vi "Append Report Text (str).vi"(0 "report in":refnum<class "NI_Standard Report.lvclass">, 1 "MS Office parameters":T1, 2 "format string (%.3f)":string="%.3f", 7 "text":string, 9 "append on new line? (F)":bool, 11 "error in (no error)":errorcluster) -> (4 "report out":refnum<class "NI_Standard Report.lvclass">, 8 "start out (Word)":i32, 10 "end out (Word)":i32, 15 "error out":errorcluster)   [LabVIEW 2015, in "NI_Standard Report.lvclass"]
doc: "Appends text to the selected report."
uses:
  <vilib>/Utility/NIReport.llb/Standard Report/NI_Standard Report.lvclass
  <vilib>/Utility/NIReport.llb/Standard Report/NI_Standard Report.lvclass/NI_Standard Report.ctl
  <vilib>/Utility/NIReport.llb/NI_ReportGenerationCore.lvlib
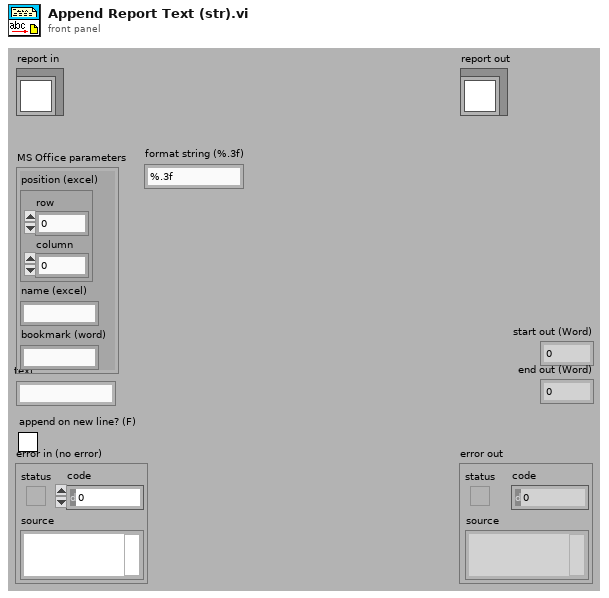
[diagram p1: front panel]
types:
  T1 = cluster{"position (excel)":cluster{"row":i32, "column":i32}, "name (excel)":string, "bookmark (word)":string}
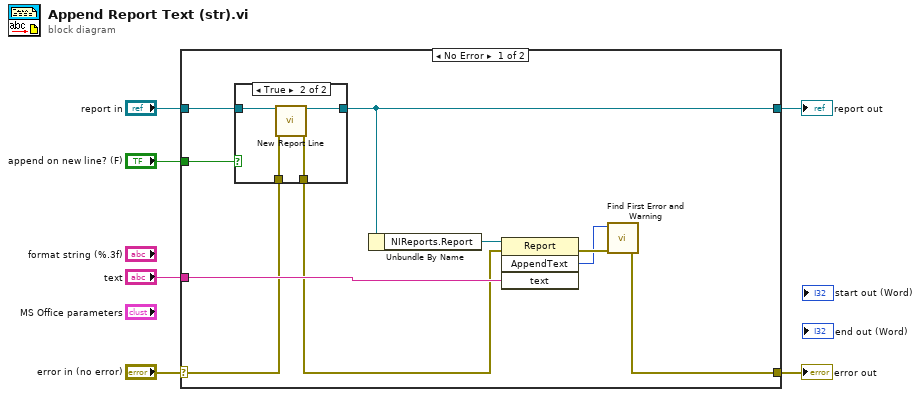
[diagram p0: block diagram]
diagram:
  n1 = case shown="No Error" "error in (no error)" {
    selector: "error in (no error)" -> [w8 w24]
    tunnel: [w9 w24] -> w5
    tunnel: [w12 w23] -> w3
    tunnel: "report in" -> [w16 w23]
    tunnel: "append on new line? (F)" -> [w15 _]
    tunnel: "text" -> [w13 _]
    frame No Error {
      n2 = case shown="True" w15 {
        tunnel: w16 -> [w18 w22]
        tunnel: [w18 w21] -> w12
        tunnel: w8 -> [w17 w20]
        tunnel: [w17 w19] -> w7
        frame False {
        }
        frame True {
          n3 = call-dynamic "New Report Line.vi"("report in"=w22, "error in (no error)"=w20) -> ("report out"=w21:refnum<class "NI_Standard Report.lvclass">, "error out"=w19:errorcluster)  [unwired: 1 in, 11 out]
        }
      }
      n4 = Unbundle By Name(w12) -> ("NIReports.Report"=w14:refnum<k7>)
      n5 = invoke class="Report" method="AppendText"(reference=w14, error in=w7, "text"=w13) -> (error out=w11:errorcluster, "AppendText"=w10:i32)  [unwired: 1 in, 2 out]
      n6 = call <vilib>:"Find First Error and Warning.vi"("error in (no error)"=w11, "error code"=w10) -> ("error out"=w9:errorcluster)  [unwired: 1 in, 4 out]
    }
    frame Error {
    }
  }
  "error out" <- w5
  "report out" <- w3
